vi "Fetch File Data.vi"(7 "File Type (0 : PNG)":i32(ring) items=["PNG (Screen Image Data)", "GNL (Setting Data)", "Other File"], 8 "error in (no error)":errorcluster, 9 "Save Path (\"\")":path, 10 "File Name (\"\")":string, 11 "VISA resource name":refnum<visa-resource-name>) -> (0 "error out":errorcluster, 3 "VISA resource name out":refnum<visa-resource-name>)   [LabVIEW 2020, in "Yokogawa GX Series.lvlib"]
doc: "Reads the data of internal memory and external medium(ex. SD card) and save to File.\n\nNote: This VI cannot save screen image data when the instrument is GM10."
uses:
  <instrlib>/Yokogawa GX Series/Yokogawa GX Series.lvlib
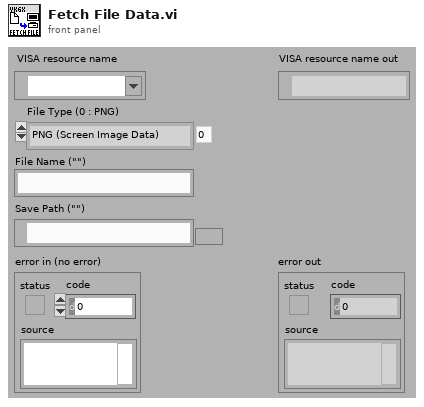
[diagram p1: front panel]
types:
  T1 = enum16{"open", "replace", "create", "open or create", "replace or create", "replace or create with confirmation"}
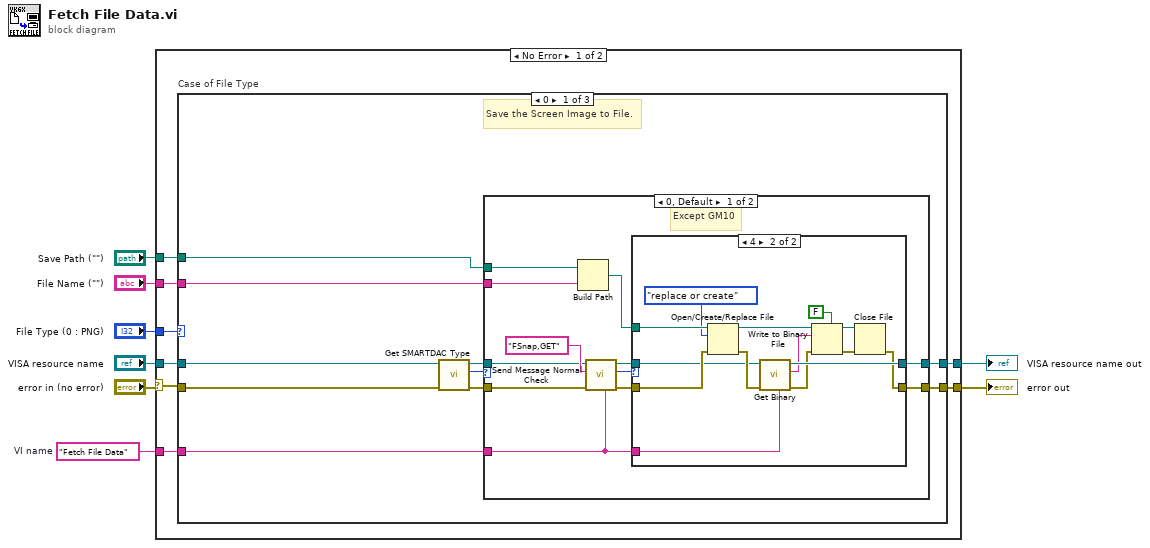
[diagram p0: block diagram]
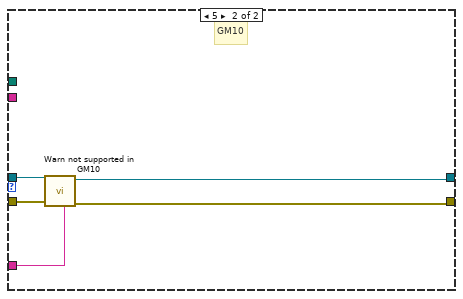
[diagram p3: hidden frame]
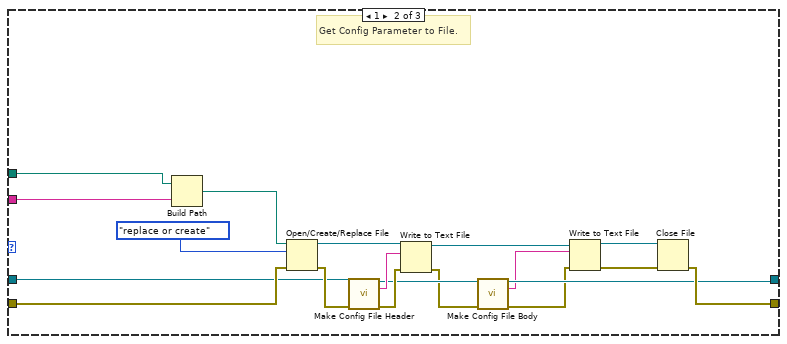
[diagram p4: hidden frame]
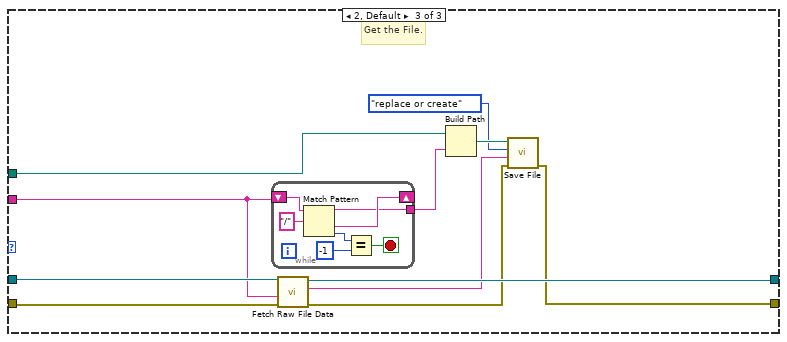
[diagram p5: hidden frame]
diagram:
  w4 = "Fetch File Data"  # VI name
  n1 = case shown="No Error" "error in (no error)" {
    selector: "error in (no error)" -> [w9 w97]
    tunnel: "Save Path (\"\")" -> [w16 _]
    tunnel: "File Name (\"\")" -> [w15 _]
    tunnel: "File Type (0 : PNG)" -> [w14 _]
    tunnel: "VISA resource name" -> [w13 w98]
    tunnel: w4 -> [w12 _]
    tunnel: [w11 w98] -> w3
    tunnel: [w10 w97] -> w2
    frame No Error {
      n2 = case "Case of File Type" shown="0" w14 {
        tunnel: w13 -> [w21 w69 w88]
        tunnel: w12 -> [w24 _ _]
        tunnel: [w25 w78 w82] -> w10
        tunnel: w9 -> [w20 w71 w87]
        tunnel: [w26 w62 w83] -> w11
        tunnel: w16 -> [w23 w77 w85]
        tunnel: w15 -> [w22 w76 w86]
        frame 0 {
          # "Save the Screen Image to File."
          n3 = call <instrlib>:"Get SMARTDAC Type.vi"("error in (no error)"=w20, "VISA resource name"=w21) -> ("error out"=w18:errorcluster, "SMARTDAC+ Type"=w17:u16, "VISA resource name out"=w19:refnum<visa-resource-name>)  [unwired: 7 in]
          n4 = case shown="0, Default" w17 {
            tunnel: [w38 w57] -> w26
            tunnel: [w37 w56] -> w25
            tunnel: w24 -> [w36 w55]
            tunnel: w23 -> [w35 _]
            tunnel: w22 -> [w34 _]
            tunnel: w19 -> [w28 w59]
            tunnel: w18 -> [w27 w58]
            frame 0, Default {
              # "Except GM10"
              n5 = Build Path(base path=w35, name or relative path=w34) -> (appended path=w33:path)
              n6 = call <instrlib>:"Send Message Normal Check.vi"("Source (\"\")"=w36, "error in (no error)"=w27, "Send Message (\"\")"="FSnap,GET", "VISA resource name"=w28) -> ("error out"=w31:errorcluster, "Response Type"=w30:i32, "VISA resource name out"=w32:refnum<visa-resource-name>)  [unwired: 1 in, 4 out]
              n7 = case shown="4" w30 {
                tunnel: w31 -> [w39 w53]
                tunnel: w32 -> [w40 w51]
                tunnel: w33 -> [_ w50]
                tunnel: [w40 w47] -> w38
                tunnel: [w39 w46] -> w37
                tunnel: w36 -> [_ w45]
                frame 0, Default {
                }
                frame 4 {
                  n8 = Open/Create/Replace File(file path (use dialog)=w50, error in=w53, operation (0:open)=T1."replace or create" ("操作（0:開く）")) -> (refnum out=w49:refnum<file>, error out=w52:errorcluster)  [unwired: 3 in, 1 out]
                  n9 = call <instrlib>:"Get Binary.vi"("Source (\"\")"=w45, "error in (no error)"=w52, "VISA resource name"=w51) -> ("error out"=w42:errorcluster, "Binary Data"=w43:string, "VISA resource name out"=w47:refnum<visa-resource-name>)  [unwired: 1 in, 5 out]
                  n10 = Write to Binary File(file (use dialog)=w49, data=w43, error in=w42, 5:FALSE ("配列または文字列サイズを先頭に追加?(T)")) -> (refnum out=w48:refnum<file>, error out=w54:errorcluster)  [unwired: 3 out]
                  n11 = Close File(refnum=w48, error in=w54) -> (error out=w46:errorcluster)  [unwired: 1 out]
                }
              }
            }
            frame 5 {
              # "GM10"
              n12 = call <instrlib>:"Warn not supported in GM10.vi"("Source (\"\")"=w55, "error in (no error)"=w58, "VISA resource name"=w59) -> ("error out"=w56:errorcluster, "VISA resource name out"=w57:refnum<visa-resource-name>)  [unwired: 7 in]
            }
          }
        }
        frame 1 {
          # "Get Config Parameter to File."
          n13 = Build Path(base path=w77, name or relative path=w76) -> (appended path=w72:path)
          n14 = Open/Create/Replace File(file path (use dialog)=w72, error in=w71, operation (0:open)=T1."replace or create" ("操作（0:開く）")) -> (refnum out=w68:refnum<file>, error out=w70:errorcluster)  [unwired: 3 in, 1 out]
          n15 = call <instrlib>:"Make Config File Header.vi"("VISA resource name"=w69, "error in (no error)"=w70) -> ("VISA resource name out"=w64:refnum<visa-resource-name>, "Result"=w67:string, "error out"=w66:errorcluster)  [unwired: 11 in]
          n16 = Write to Text File(file (use dialog)=w68, text=w67, error in=w66) -> (refnum out=w65:refnum<file>, error out=w63:errorcluster)  [unwired: 1 in, 1 out]
          n17 = call <instrlib>:"Make Config File Body.vi"("VISA resource name"=w64, "error in (no error)"=w63) -> ("VISA resource name out"=w62:refnum<visa-resource-name>, "Result"=w60:string, "error out"=w61:errorcluster)  [unwired: 11 in]
          n18 = Write to Text File(file (use dialog)=w65, text=w60, error in=w61) -> (refnum out=w74:refnum<file>, error out=w75:errorcluster)  [unwired: 1 in, 1 out]
          n19 = Close File(refnum=w74, error in=w75) -> (error out=w78:errorcluster)  [unwired: 1 out]
        }
        frame 2, Default {
          # "Get the File."
          n20 = while {
            shift-right: [w94] -> _
            shift-left: w86 -> [w96]
            tunnel: [w90] -> w89
            stop <- w91 stop-if-true
            n21 = Match Pattern(string=w96, regular expression="/" ("正規表現")) -> (before substring=w90:string, after substring=w94:string, offset past match=w93:i32)  [unwired: 2 out]
            n22 = Equal?(x=w93, y=-1 ("一致後オフセット")) -> (x = y?=w91:bool)
          }
          n23 = call <instrlib>:"Fetch Raw File Data.vi"("error in (no error)"=w87, "Read File Name (\"\")"=w86, "VISA resource name"=w88) -> ("error out"=w80:errorcluster, "Data"=w81:string, "VISA resource name out"=w83:refnum<visa-resource-name>)  [unwired: 6 in]
          n24 = Build Path(base path=w85, name or relative path=w89) -> (appended path=w84:path)
          n25 = call <instrlib>:"Save File.vi"("error in (no error)"=w80, "Data (\"\")"=w81, "Operation (0 : Open)"=T1."replace or create" ("操作（0:開く）"), "File Path (\"\")"=w84) -> ("error out"=w82:errorcluster)  [unwired: 7 in]
        }
      }
    }
    frame Error {
    }
  }
  "error out" <- w2
  "VISA resource name out" <- w3
